vi "Banks to Modules.vi"(8 "error in (no error)":errorcluster, 11 "SL_SC in":refnum<class "SL_SC.lvclass">) -> (0 "error out":errorcluster, 3 "SL_SC out":refnum<class "SL_SC.lvclass">)   [LabVIEW 2019, in "SL_SC.lvlib" / "SL_SC.lvclass"]
uses:
  Library/SL_SC.lvclass
  C:/Users/Public/Documents/Development/builds/Instruments/DIG_IO.lvlibp/Library/DIG_IO.lvclass
  builds/Instruments/DIG_IO.lvlibp/Accessors/Read Banks.vi
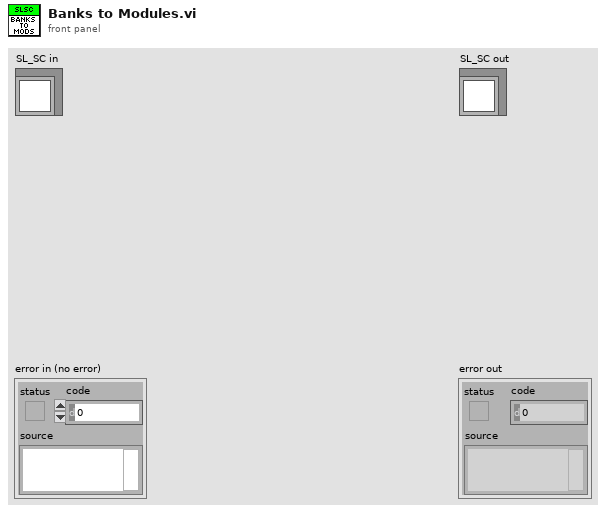
[diagram p1: front panel]
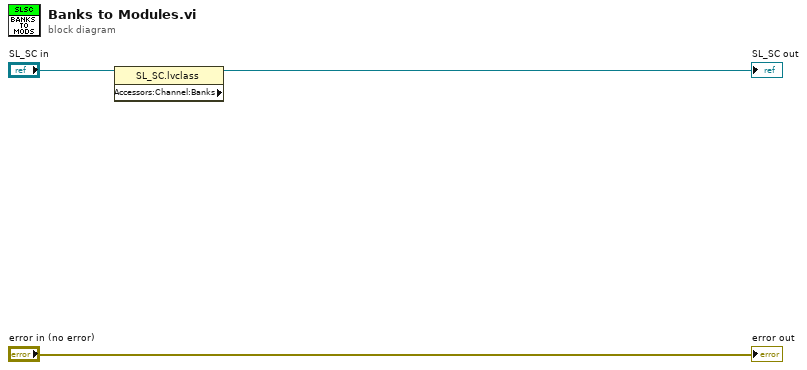
[diagram p0: block diagram]
diagram:
  n1 = property class="SL_SC.lvclass" props=["Accessors:Channel:Banks"](reference="SL_SC in") -> (reference out=→"SL_SC out":refnum<class "SL_SC.lvclass">)  [unwired: 1 in, 2 out]
  "error out" <- "error in (no error)"
